vi "testing.vi"() -> ()   [LabVIEW 2011]
uses:
  <vilib>/regexp/Match Regular Expression.xnode
panel:
  out "whole match 2":string
  in  "regular expression 2":string
  out "after match":string
  out "whole match":string
  out "before match":string
  in  "input string":string
  in  "regular expression":string
  in  "stop":bool
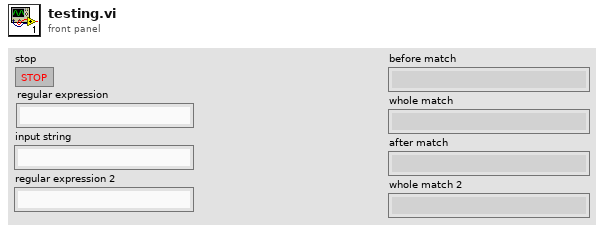
[diagram p1: front panel]
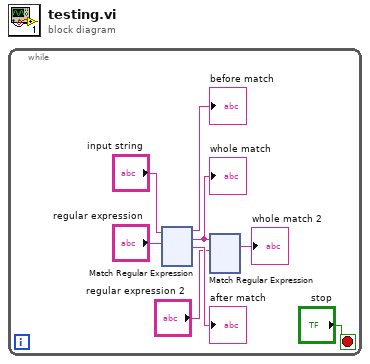
[diagram p0: block diagram]
diagram:
  n1 = while {
    stop <- "stop" stop-if-true
    n2 = xnode "Match Regular Expression"("input string"="input string", "regular expression"="regular expression") -> ("before match"=→"before match":string, "whole match"=w1:string, "after match"=→"after match":string)  [unwired: 4 in, 2 out]
    "whole match" <- w1
    n3 = xnode "Match Regular Expression"("input string"=w1, "regular expression"="regular expression 2") -> ("whole match"=→"whole match 2":string)  [unwired: 4 in, 4 out]
  }
